vi "PID_lead_lag.vi"(8 "dt (s) in":dbl=-1.0, 10 "Tuning parameters":T1={"Gain"=0.0, "Lag time"=0.01, "Lead Time"=0.0} {"Lead Time" format="%_6g"; "Lag time" format="%_6g"; "Gain" format="%_6g"}, 11 "Input":dbl) -> (3 "Output":dbl format="%_6g")   [LabVIEW 2010]
panel:
  in  "Output Rnage":cluster{"output high":dbl, "output low":dbl}={"output high"=100.0, "output low"=-100.0}
  in  "reinitialize?":bool
  out "dt (s) out":dbl format="%_6g"
  in  "Time unit":u16(ring) items=["Second", "Minute"]
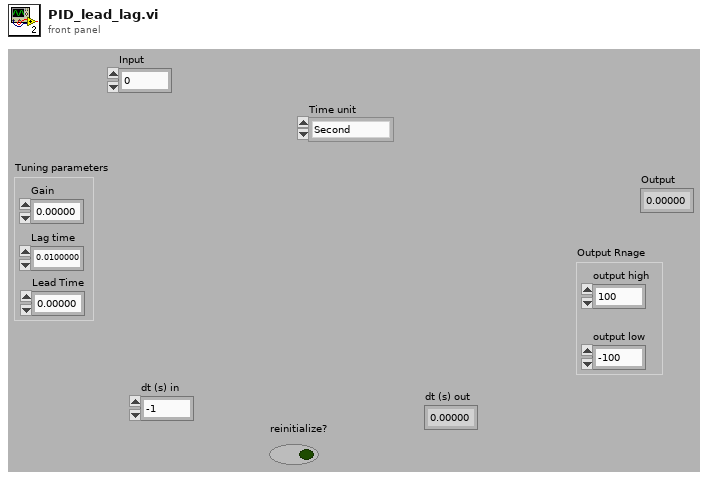
[diagram p1: front panel]
types:
  T1 = cluster{"Gain":dbl, "Lag time":dbl, "Lead Time":dbl}
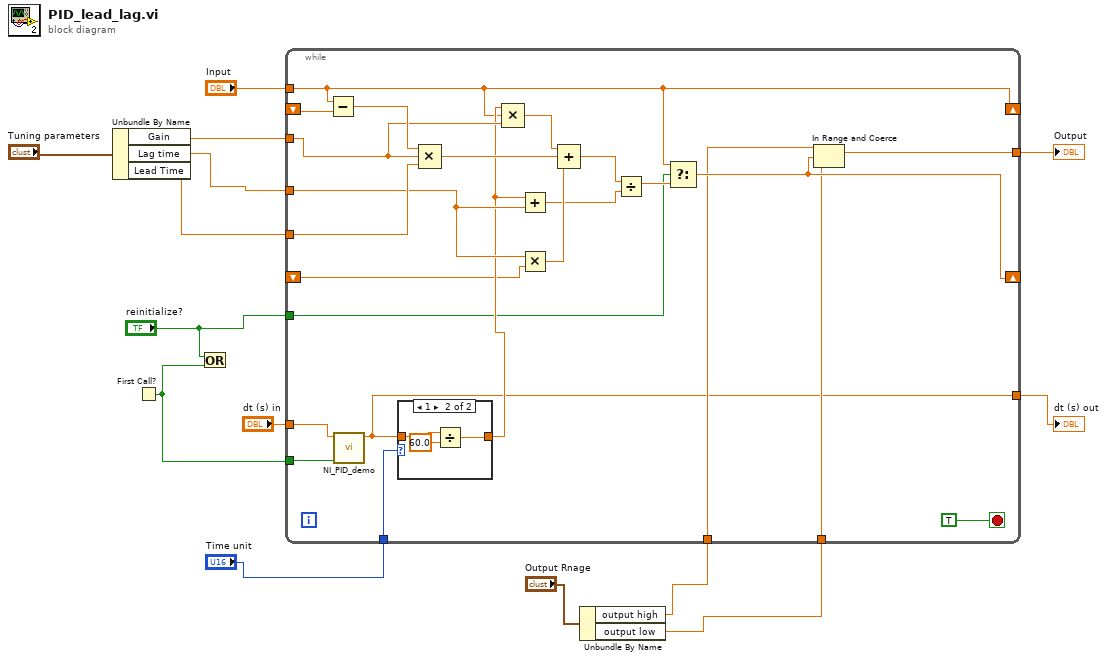
[diagram p0: block diagram]
diagram:
  n1 = Unbundle By Name("Tuning parameters") -> ("Gain"=w6:dbl, "Lag time"=w5:dbl, "Lead Time"=w4:dbl)
  n2 = First Call?() -> (First Call?: T/F=w11:bool)
  n3 = Or(x="reinitialize?", y=w11) -> ()  [unwired: 1 out]
  n4 = Unbundle By Name("Output Rnage") -> ("output high"=w2:dbl, "output low"=w1:dbl)
  n5 = while {
    shift-right: [w21] -> _
    shift-left: _ -> [w37]
    tunnel: "Input" -> [w21]
    tunnel: w6 -> [w31]
    tunnel: w4 -> [w35]
    tunnel: "Time unit" -> [w34]
    tunnel: "dt (s) in" -> [w33]
    tunnel: w11 -> [w32]
    tunnel: w5 -> [w28]
    shift-right: [w19] -> _
    shift-left: _ -> [w26]
    tunnel: "reinitialize?" -> [w20]
    tunnel: w2 -> [w18]
    tunnel: w1 -> [w17]
    tunnel: [w16] -> w9
    tunnel: [w15] -> w8
    stop <- TRUE stop-if-true
    n6 = Subtract(x=w21, y=w37) -> (x-y=w36:dbl)
    n7 = call "NI_PID_demo.vi"("Initialize"=w32, "dt (s) in"=w33) -> ("dt (s) out"=w15:dbl)  [unwired: 9 in]
    n8 = case shown="1" w34 {
      tunnel: w15 -> [w39 w42]
      tunnel: [w39 w41] -> w27
      frame 0, Default {
      }
      frame 1 {
        n9 = Divide(x=w42, y=60.0) -> (x/y=w41:dbl)
      }
    }
    n10 = Compound Arithmetic op=MULTIPLY(w36, w31, w35) -> (w29:dbl)
    n11 = Compound Arithmetic op=MULTIPLY(w27, w21, w31) -> (w30:dbl)
    n12 = Add(x=w27, y=w28) -> (x+y=w23:dbl)
    n13 = Multiply(x=w28, y=w26) -> (x*y=w25:dbl)
    n14 = Compound Arithmetic op=ADD(w30, w29, w25) -> (w24:dbl)
    n15 = Divide(x=w24, y=w23) -> (x/y=w22:dbl)
    n16 = Select(t=w21, s=w20, f=w22) -> (s? t:f=w19:dbl)
    n17 = In Range and Coerce(upper limit=w18, x=w19, lower limit=w17) -> (coerced(x)=w16:dbl)  [unwired: 1 out]
  }
  "Output" <- w9
  "dt (s) out" <- w8
